vi "GenerateCode.vi"(0 "XRef":T17, 1 "Terms":T14, 2 "Diagram":T13, 3 "State In":T1) -> (14 "Generated Code?":T9, 15 "Reply":T12, 16 "Fatal Error Out":T11, 17 "State Out":T1)   [LabVIEW 2021, in "myRIO Encoder Open.xnode"]
uses:
  <vilib>/myRIO/Instrument Drivers/Onboard IO/Encoder/vis/myRIO Encoder Open.xnode
  <vilib>/XNodeSupport/XNodeXNodeRef.ctl
  <vilib>/XNodeSupport/XNodeTermIDPairs.ctl
  <vilib>/XNodeSupport/XNodeTermIDPair.ctl
  <vilib>/XNodeSupport/XNodeTermRef.ctl
  <vilib>/XNodeSupport/XNodeString.ctl
  <vilib>/XNodeSupport/XNodeTopLevelDiagramRef.ctl
  <vilib>/myRIO/Instrument Drivers/Onboard IO/Encoder/vis/State.ctl
  <vilib>/myRIO/Common/Instrument Driver Framework/Utilities/typedefs/myRIOXPeripheral.ctl
  <vilib>/XNodeSupport/XNodeTerm4Array.ctl
  <vilib>/XNodeSupport/XNodeTerm4.ctl
  <vilib>/XNodeSupport/XNodeVariant.ctl
  <vilib>/XNodeSupport/XNodeRect32.ctl
  <vilib>/XNodeSupport/XNodeInt.ctl
  <vilib>/XNodeSupport/XNodeBool.ctl
  <vilib>/XNodeSupport/XNodeTermDirection.ctl
  <vilib>/XNodeSupport/XNodeStringArray.ctl
  <vilib>/XNodeSupport/XNodeErrorCluster.ctl
  <vilib>/Utility/miscctls.llb/LVPositionTypeDef.ctl
  <vilib>/Utility/miscctls.llb/LVPointTypeDef.ctl
  <vilib>/userdefined/High Color/nirio_resource_hc.ctl
  <vilib>/XNodeSupport/NI_XNodeSupport.lvlib
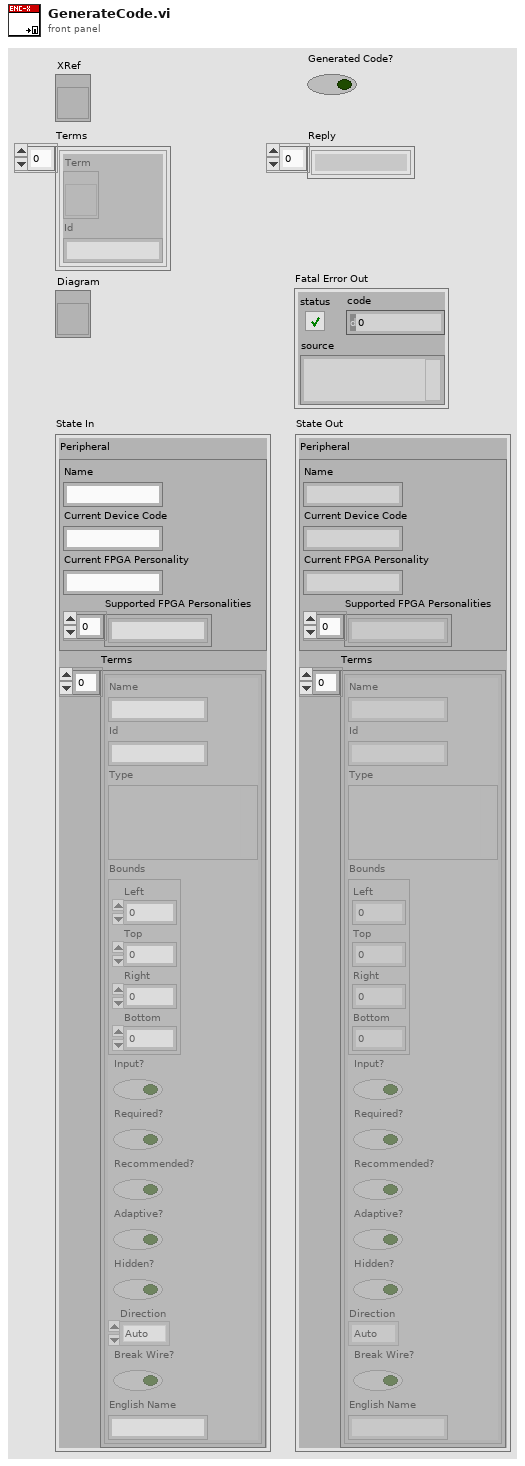
[diagram p1: front panel]
types:
  T1 = typedef "myRIO Encoder Open.xnode/State.ctl" = cluster{"Peripheral":T2, "Terms":T3}
  T2 = typedef "myRIOXPeripheral.ctl" = cluster{"Name":string, "Current Device Code":string, "Current FPGA Personality":string, "Supported FPGA Personalities":string[]}
  T3 = typedef "NI_XNodeSupport.lvlib/XNodeTerm4Array.ctl" = T4[]
  T4 = typedef "NI_XNodeSupport.lvlib/XNodeTerm4.ctl" = cluster{"Name":T5, "Id":T5, "Type":T6, "Bounds":T7, "Input?":T9, "Required?":T9, "Recommended?":T9, "Adaptive?":T9, "Hidden?":T9, "Direction":T10, "Break Wire?":T9, "English Name":T5}
  T5 = typedef "NI_XNodeSupport.lvlib/XNodeString.ctl" = string
  T6 = typedef "NI_XNodeSupport.lvlib/XNodeVariant.ctl" = variant
  T7 = typedef "NI_XNodeSupport.lvlib/XNodeRect32.ctl" = cluster{"Left":T8, "Top":T8, "Right":T8, "Bottom":T8}
  T8 = typedef "NI_XNodeSupport.lvlib/XNodeInt.ctl" = i32
  T9 = typedef "NI_XNodeSupport.lvlib/XNodeBool.ctl" = bool
  T10 = typedef "NI_XNodeSupport.lvlib/XNodeTermDirection.ctl" = enum32{"Auto", "Up", "Down", "Left", "Right", "Center"}
  T11 = typedef "NI_XNodeSupport.lvlib/XNodeErrorCluster.ctl" = errorcluster
  T12 = typedef "NI_XNodeSupport.lvlib/XNodeStringArray.ctl" = T5[]
  T13 = typedef "NI_XNodeSupport.lvlib/XNodeTopLevelDiagramRef.ctl" = refnum<vi>
  T14 = typedef "NI_XNodeSupport.lvlib/XNodeTermIDPairs.ctl" = T15[]
  T15 = typedef "NI_XNodeSupport.lvlib/XNodeTermIDPair.ctl" = cluster{"Term":T16, "Id":T5}
  T16 = typedef "NI_XNodeSupport.lvlib/XNodeTermRef.ctl" = refnum<vi>
  T17 = typedef "NI_XNodeSupport.lvlib/XNodeXNodeRef.ctl" = refnum<vi>
  T18 = typedef "LVPositionTypeDef.ctl" = cluster{"Left":i32, "Top":i32}
  T19 = typedef "LVPointTypeDef.ctl" = cluster{"Horizontal":i16, "Vertical":i16}
  T20 = typedef "nirio_resource_hc.ctl" = tag
  T21 = typedef "Hardware Version Enum.ctl" = enum16{"Unknown", "myRIO-1900", "myRIO-1950", "roboRIO", "NI ELVIS RIO CM", "ELVIS III"}
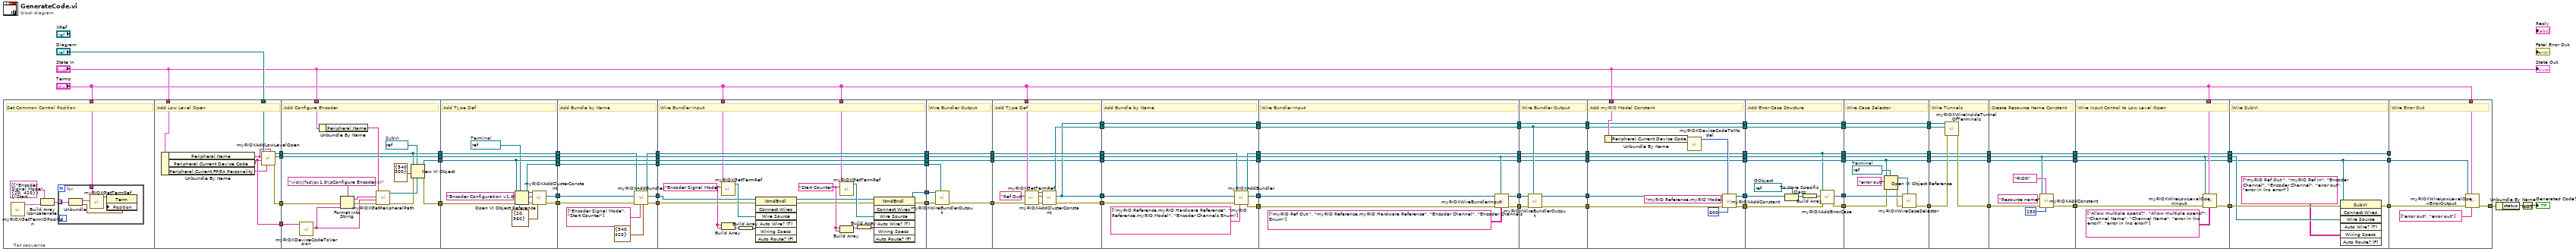
[diagram p0: block diagram]
diagram:
  n1 = flat-sequence {
    tunnel: "Terms" -> [w103]
    tunnel: "State In" -> [w116]
    tunnel: "Diagram" -> [w115]
    tunnel: [w114] -> w55
    tunnel: [w113] -> w54
    tunnel: [w111] -> w53
    tunnel: [w110] -> w1
    tunnel: w55 -> [w123]
    tunnel: [w123] -> w50
    tunnel: w54 -> [w131]
    tunnel: [w131] -> w49
    tunnel: [w128] -> w48
    tunnel: w53 -> [w119]
    tunnel: "State In" -> [w126]
    tunnel: [w124] -> w47
    tunnel: w1 -> [w120]
    tunnel: w50 -> [w143]
    tunnel: [w143] -> w46
    tunnel: w49 -> [w142]
    tunnel: [w142] -> w45
    tunnel: w48 -> [w139]
    tunnel: [w135] -> w44
    tunnel: w47 -> [w141]
    tunnel: [w141] -> w43
    tunnel: [w134] -> w42
    tunnel: [w138] -> w26
    tunnel: w46 -> [w148]
    tunnel: [w147] -> w41
    tunnel: w45 -> [w154]
    tunnel: [w154] -> w40
    tunnel: w44 -> [w151]
    tunnel: [w150] -> w39
    tunnel: w43 -> [w153]
    tunnel: [w153] -> w38
    tunnel: w42 -> [w149]
    tunnel: [w146] -> w37
    tunnel: w26 -> [w145]
    tunnel: [w145] -> w24
    tunnel: w41 -> [w174]
    tunnel: [w174] -> w35
    tunnel: w40 -> [w173]
    tunnel: [w173] -> w33
    tunnel: w39 -> [w170]
    tunnel: [w164] -> w31
    tunnel: w38 -> [w172]
    tunnel: [w172] -> w29
    tunnel: w37 -> [w171]
    tunnel: "Terms" -> [w169]
    tunnel: "Terms" -> [w163]
    tunnel: [w156] -> w27
    tunnel: [w155] -> w25
    tunnel: w24 -> [w155]
    tunnel: w35 -> [w181]
    tunnel: [w181] -> w34
    tunnel: w33 -> [w180]
    tunnel: [w180] -> w32
    tunnel: w31 -> [w178]
    tunnel: [w177] -> w30
    tunnel: w29 -> [w179]
    tunnel: [w179] -> w28
    tunnel: w27 -> [w176]
    tunnel: w25 -> [w175]
    tunnel: "Terms" -> [w192]
    tunnel: [w186] -> w99
    tunnel: [w189] -> w98
    tunnel: w34 -> [w189]
    tunnel: [w188] -> w95
    tunnel: w32 -> [w188]
    tunnel: [w187] -> w91
    tunnel: [w186] -> w86
    tunnel: [w185] -> w65
    tunnel: w30 -> [w183]
    tunnel: [w182] -> w51
    tunnel: w28 -> [w182]
    tunnel: w99 -> [w203]
    tunnel: w98 -> [w200]
    tunnel: [w202] -> w97
    tunnel: [w201] -> w96
    tunnel: w95 -> [w201]
    tunnel: [w199] -> w93
    tunnel: w91 -> [w198]
    tunnel: [w198] -> w89
    tunnel: [w197] -> w87
    tunnel: w86 -> [w197]
    tunnel: w65 -> [w196]
    tunnel: [w195] -> w64
    tunnel: w51 -> [w193]
    tunnel: [w193] -> w23
    tunnel: w97 -> [w213]
    tunnel: w96 -> [w208]
    tunnel: [w212] -> w85
    tunnel: [w211] -> w83
    tunnel: w93 -> [w211]
    tunnel: [w210] -> w81
    tunnel: w89 -> [w210]
    tunnel: [w209] -> w79
    tunnel: w87 -> [w209]
    tunnel: [w208] -> w76
    tunnel: w64 -> [w207]
    tunnel: [w206] -> w63
    tunnel: w23 -> [w204]
    tunnel: [w204] -> w19
    tunnel: w85 -> [w222]
    tunnel: [w219] -> w84
    tunnel: w83 -> [w221]
    tunnel: [w221] -> w82
    tunnel: w81 -> [w218]
    tunnel: [w218] -> w80
    tunnel: w79 -> [w220]
    tunnel: [w220] -> w78
    tunnel: [w217] -> w77
    tunnel: w76 -> [w217]
    tunnel: w63 -> [w216]
    tunnel: [w215] -> w62
    tunnel: [w214] -> w20
    tunnel: w19 -> [w214]
    tunnel: w84 -> [w236]
    tunnel: "State In" -> [w234]
    tunnel: [w230] -> w94
    tunnel: w82 -> [w230]
    tunnel: [w229] -> w92
    tunnel: [w228] -> w90
    tunnel: w80 -> [w228]
    tunnel: [w227] -> w88
    tunnel: w78 -> [w227]
    tunnel: w77 -> [w226]
    tunnel: [w226] -> w74
    tunnel: w62 -> [w225]
    tunnel: [w224] -> w61
    tunnel: [w223] -> w21
    tunnel: w20 -> [w223]
    tunnel: w94 -> [w237]
    tunnel: w92 -> [w248]
    tunnel: [w244] -> w72
    tunnel: w90 -> [w244]
    tunnel: [w243] -> w70
    tunnel: w88 -> [w243]
    tunnel: [w242] -> w68
    tunnel: w74 -> [w242]
    tunnel: [w241] -> w66
    tunnel: w61 -> [w240]
    tunnel: [w239] -> w60
    tunnel: [w238] -> w22
    tunnel: w21 -> [w238]
    tunnel: [w237] -> w6
    tunnel: w72 -> [w260]
    tunnel: [w260] -> w71
    tunnel: w70 -> [w259]
    tunnel: [w259] -> w69
    tunnel: w68 -> [w255]
    tunnel: [w255] -> w67
    tunnel: w66 -> [w258]
    tunnel: w60 -> [w251]
    tunnel: [w253] -> w59
    tunnel: w22 -> [w250]
    tunnel: [w250] -> w16
    tunnel: [w249] -> w7
    tunnel: w6 -> [w249]
    tunnel: w71 -> [w266]
    tunnel: w69 -> [w267]
    tunnel: [w265] -> w75
    tunnel: w67 -> [w265]
    tunnel: w59 -> [w264]
    tunnel: [w263] -> w58
    tunnel: [w262] -> w17
    tunnel: w16 -> [w262]
    tunnel: [w261] -> w8
    tunnel: w7 -> [w261]
    tunnel: w75 -> [w272]
    tunnel: [w272] -> w73
    tunnel: w58 -> [w271]
    tunnel: [w270] -> w57
    tunnel: [w269] -> w18
    tunnel: w17 -> [w269]
    tunnel: [w268] -> w9
    tunnel: w8 -> [w268]
    tunnel: w73 -> [w277]
    tunnel: "Terms" -> [w281]
    tunnel: [w280] -> w15
    tunnel: w57 -> [w279]
    tunnel: [w278] -> w13
    tunnel: w18 -> [w278]
    tunnel: [w277] -> w11
    tunnel: [w276] -> w10
    tunnel: w9 -> [w276]
    tunnel: w15 -> [w288]
    tunnel: [w287] -> w14
    tunnel: w13 -> [w285]
    tunnel: [w285] -> w12
    tunnel: w11 -> [w286]
    tunnel: w10 -> [w283]
    tunnel: [w283] -> w5
    tunnel: [w292] -> w4
    tunnel: w14 -> [w293]
    tunnel: "Terms" -> [w291]
    tunnel: w12 -> [w289]
    tunnel: w5 -> [_]
    frame #0 {
      # "Set Common Control Position"
      n2 = call <vilib>:"myRIOXGetTermIDPosition.vi"() -> ("Term ID Postion"=w102:cluster{"Term ID":string, "Position":T18}[])  [unwired: 11 in]
      n3 = Build Array (concatenate)(cluster{"Term ID":string, "Position":T18}[] [{"Term ID"="Encoder Signal Mode", "Position"={"Left"=20, "Top"=420}}, {"Term ID"="Start Counter", "Position"={"Left"=20, "Top"=450}}] ("array"), w102) -> (w101:cluster{"Term ID":string, "Position":T18}[])
      n4 = for {
        tunnel: w103 -> [w108]
        tunnel: w101 -> [w106] mode=indexing
        n5 = Unbundle(w106) -> ("Term ID"=w105:string, "Position"=w104:T18)
        n6 = call <vilib>:"myRIOXGetTermRef.vi"("Term ID"=w105, "Terms"=w108) -> ("Terminal Reference"=w107:T16)  [unwired: 7 in, 2 out]
        n7 = property class="Term"(reference=w107, "Position"=w104) -> ()  [unwired: 1 in, 2 out]
      }
    }
    frame #1 {
      # "Add Low Level Open"
      n8 = Unbundle By Name(w116) -> ("Peripheral.Name"=w109:string, "Peripheral.Current Device Code"=w110:string, "Peripheral.Current FPGA Personality"=w112:string)
      n9 = call <vilib>:"myRIOXAddLowLevelOpen.vi"("Peripheral Name"=w109, "FPGA Personality"=w112, "Device Code"=w110, "VI Name"=w109, "Diagram Reference"=w115) -> ("error out"=w111:errorcluster, "SubVI Reference"=w113:refnum<vi>, "Duplicated Diagram Reference"=w114:T13)  [unwired: 4 in]
    }
    frame #2 {
      w129 = refnum<vi> refnum  # SubVI
      # "Add Configure Encoder"
      n10 = call <vilib>:"myRIOXDeviceCodeToVersion.vi"("Device Code"=w120) -> ("Name"=w117:string)  [unwired: 9 in, 1 out]
      n11 = Unbundle By Name(w126) -> ("Peripheral.Name"=w125:string)
      n12 = Format Into String(format string="vis\\\\%s\\sv1.0\\sConfigure Encoder.vi", error in=w119, w117) -> (resulting string=w121:string, error out=w118:errorcluster)  [unwired: 1 in]
      n13 = call <vilib>:"myRIOXGetPeripheralPath.vi"("error in (no error)"=w118, "Device Name"=w117, "VI Name"=w121, "Peripheral Name"=w125) -> ("error out"=w127:errorcluster, "Peripheral Path"=w130:path)  [unwired: 6 in]
      n14 = New VI Object(vi object class=w129, owner refnum=w123, position/next to=T19 {"Horizontal"=540, "Vertical"=300} ("location"), 6:w130, 8:w127) -> (object refnum=w124:refnum<vi>, 0:w128:errorcluster)  [unwired: 3 in]
    }
    frame #3 {
      w140 = refnum<vi> refnum  # Terminal
      w136 = "Encoder Configuration v1.0" ("name/order")
      # "Add Type Def"
      n15 = Open VI Object Reference(7:w140, 8:w139, 10:w136, 11:w141) -> (0:w137:errorcluster, 3:w138:refnum<vi>)
      n16 = call <vilib>:"myRIOXAddClusterConstant.vi"("Position (20,90)"=T18 {"Left"=20, "Top"=360} ("Position"), "error in (no error)"=w137, "Full Term ID"=w136, "Term Reference"=w138) -> ("error out"=w135:errorcluster, "Cluster Constant Terminal Reference"=w134:refnum<vi>)  [unwired: 5 in, 1 out]
    }
    frame #4 {
      # "Add Bundle by Name"
      n17 = call <vilib>:"myRIOXAddBundler.vi"("Position (770,158)"=T18 {"Left"=340, "Top"=420}, "Element Names"=string[] ["Encoder Signal Mode", "Start Counter"], "error in (no error)"=w151, "Cluster Constant Terminal Reference"=w149, "Diagram Reference"=w148) -> ("error out"=w150:errorcluster, "Named Bundler Reference"=w146:refnum<vi>, "Duplicated Diagram Reference"=w147:T13)  [unwired: 4 in]
    }
    frame #5 {
      w159 = "Start Counter" ("Term ID")
      w162 = "Encoder Signal Mode" ("Term ID")
      # "Wire Bundler Input"
      n18 = call <vilib>:"myRIOXGetTermRef.vi"("Term ID"=w162, "Terms"=w169) -> ("Terminal Reference"=w168:T16)  [unwired: 7 in, 2 out]
      n19 = Build Array(w162, w162) -> (w161:string[])
      n20 = Build Array(w161) -> (w160:string[][])
      n21 = invoke class="NmdBndl" method="Connect Wires"(reference=w171, error in=w170, "Wire Source"=w168, "Wiring Specs"=w160) -> (reference out=w165:refnum<vi>, error out=w166:errorcluster)  [unwired: 3 in, 5 out]
      n22 = call <vilib>:"myRIOXGetTermRef.vi"("Term ID"=w159, "Terms"=w163) -> ("Terminal Reference"=w167:T16)  [unwired: 7 in, 2 out]
      n23 = Build Array(w159, w159) -> (w158:string[])
      n24 = Build Array(w158) -> (w157:string[][])
      n25 = invoke class="NmdBndl" method="Connect Wires"(reference=w165, error in=w166, "Wire Source"=w167, "Wiring Specs"=w157) -> (reference out=w156:refnum<vi>, error out=w164:errorcluster)  [unwired: 3 in, 5 out]
    }
    frame #6 {
      # "Wire Bundler Output"
      n26 = call <vilib>:"myRIOXWireBundlerOutput.vi"("Sink Terminam Reference"=w175, "error in (no error)"=w178, "Named Bundler Reference"=w176) -> ("error out"=w177:errorcluster)  [unwired: 7 in, 1 out]
    }
    frame #7 {
      # "Add Type Def"
      n27 = call <vilib>:"myRIOXGetTermRef.vi"("Term ID"="Ref Out", "Terms"=w192) -> ("Full Term ID"=w190:T5, "Terminal Reference"=w184:T16)  [unwired: 7 in, 1 out]
      n28 = call <vilib>:"myRIOXAddClusterConstant.vi"("error in (no error)"=w183, "Full Term ID"=w190, "Term Reference"=w184) -> ("error out"=w185:errorcluster, "Cluster Constant Terminal Reference"=w186:refnum<vi>, "Duplicated Term Reference"=w187:T16)  [unwired: 6 in]
    }
    frame #8 {
      # "Add Bundle by Name"
      n29 = call <vilib>:"myRIOXAddBundler.vi"("Element Names"=string[] ["myRIO Reference.myRIO Hardware Reference", "myRIO Reference.myRIO Model", "Encoder Channels Enum"], "error in (no error)"=w196, "Cluster Constant Terminal Reference"=w203, "Diagram Reference"=w200) -> ("error out"=w195:errorcluster, "Named Bundler Reference"=w202:refnum<vi>, "Duplicated Diagram Reference"=w199:T13)  [unwired: 5 in]
    }
    frame #9 {
      # "Wire Bundler Input"
      n30 = call <vilib>:"myRIOXWireBundlerInput.vi"("Wiring Specs"=string[][] [["myRIO Ref Out ", "myRIO Reference.myRIO Hardware Reference"], ["Encoder Channel", "Encoder Channels Enum"]], "SubVI Reference"=w208, "error in (no error)"=w207, "Named Bundler Reference"=w213) -> ("error out"=w206:errorcluster, "Duplicated Named Bundler Reference"=w212:refnum<vi>)  [unwired: 6 in]
    }
    frame #10 {
      # "Wire Bundler Output"
      n31 = call <vilib>:"myRIOXWireBundlerOutput.vi"("Sink Terminam Reference"=w218, "error in (no error)"=w216, "Named Bundler Reference"=w222) -> ("error out"=w215:errorcluster, "Duplicated Named Bundler Reference"=w219:refnum<vi>)  [unwired: 7 in]
    }
    frame #11 {
      # "Add myRIO Model Constant"
      n32 = Unbundle By Name(w234) -> ("Peripheral.Current Device Code"=w233:string)
      n33 = call <vilib>:"myRIOXDeviceCodeToModel.vi"("Device Code"=w233) -> ("myRIO Reference.myRIO Model"=w232:T21)  [unwired: 10 in]
      n34 = call <vilib>:"myRIOXAddConstant.vi"("Left (0)"=600 ("Left"), "Value"=w232, "error in (no error)"=w225, "Terminal Name"="myRIO Reference.myRIO Model", "Owner Reference"=w236) -> ("error out"=w224:errorcluster, "Duplicated Owner Reference"=w229:refnum<vi>)  [unwired: 5 in]
    }
    frame #12 {
      w245 = refnum<vi> refnum  # GObject
      # "Add Error Case Structure"
      n35 = To More Specific Class(target class=w245, reference=w248) -> (specific class reference=w246:refnum<vi>)  [unwired: 1 in, 1 out]
      n36 = Build Array(w246) -> (w247:refnum<vi>[])
      n37 = call <vilib>:"myRIOXAddErrorCase.vi"("error in (no error)"=w240, "Enclosed Object References"=w247, "Diagram Reference"=w237) -> ("error out"=w239:errorcluster, "Case Structure Reference"=w241:refnum<vi>)  [unwired: 6 in, 1 out]
    }
    frame #13 {
      w257 = refnum<vi> refnum  # Terminal
      # "Wire Case Selector"
      n38 = Open VI Object Reference(7:w257, 8:w251, 10:"error out" ("name/order"), 11:w250) -> (0:w252:errorcluster, 3:w256:refnum<vi>)
      n39 = call <vilib>:"myRIOXWireCaseSelector.vi"("Source Terminam Reference"=w256, "error in (no error)"=w252, "Case Structure Reference"=w258) -> ("error out"=w253:errorcluster)  [unwired: 7 in, 1 out]
    }
    frame #14 {
      # "Wire Tunnels"
      n40 = call <vilib>:"myRIOXWireInsideTunnelOfTerminals.vi"("error in (no error)"=w264, "Sink Terminam Reference"=w266, "Source Terminam Reference"=w267) -> ("error out"=w263:errorcluster)  [unwired: 6 in, 2 out]
    }
    frame #15 {
      # "Create Resource Name Constant"
      n41 = call <vilib>:"myRIOXAddConstant.vi"("Left (0)"=250 ("Left"), "Value"=T20 "RIO0" ("Resource name"), "error in (no error)"=w271, "Terminal Name"="Resource name", "Owner Reference"=w272) -> ("error out"=w270:errorcluster)  [unwired: 5 in, 1 out]
    }
    frame #16 {
      # "Wire Input Control to Low Level Open"
      n42 = call <vilib>:"myRIOXWireLowLevelOpenInput.vi"("Wiring Specs"=string[][] [["Allow multiple opens?", "Allow multiple opens?"], ["Channel Name", "Channel Name"], ["error in (no error)", "error in (no error)"]], "Terms"=w281, "error in (no error)"=w279, "SubVI Reference"=w277) -> ("error out"=w280:errorcluster)  [unwired: 6 in, 1 out]
    }
    frame #17 {
      # "Wire SubVI"
      n43 = invoke class="SubVI" method="Connect Wires"(reference=w285, error in=w288, "Wire Source"=w286, "Wiring Specs"=string[][] [["myRIO Ref Out ", "myRIO Ref In"], ["Encoder Channel", "Encoder Channel"], ["error out", "error in (no error)"]]) -> (error out=w287:errorcluster)  [unwired: 3 in, 6 out]
    }
    frame #18 {
      # "Wire Error Out"
      n44 = call <vilib>:"myRIOXWireLowLevelOpenErrorOutput.vi"("Wiring Specs"=string[] ["error out", "error out"], "Terms"=w291, "error in (no error)"=w293, "SubVI Reference"=w289) -> ("error out"=w292:errorcluster)  [unwired: 6 in, 1 out]
    }
  }
  n45 = Unbundle By Name(w4) -> ("status"=w3:bool)
  n46 = Not(x=w3) -> (.not. x?=→"Generated Code?":bool)
  "State Out" <- "State In"
